vi "USB2XXXSPISlaveContinueReadTest.vi"() -> ()   [LabVIEW 2010]
panel:
  in  "stop":bool
  out "Read Data(Hex)":string
  in  "pConfig":T1
  in  "Channel Index":i32(ring) items=["SPI1_CS0", "SPI2_CS0"]
  in  "Device Index":i32(ring) items=["0", "1", "2", "3", "4", "5"]
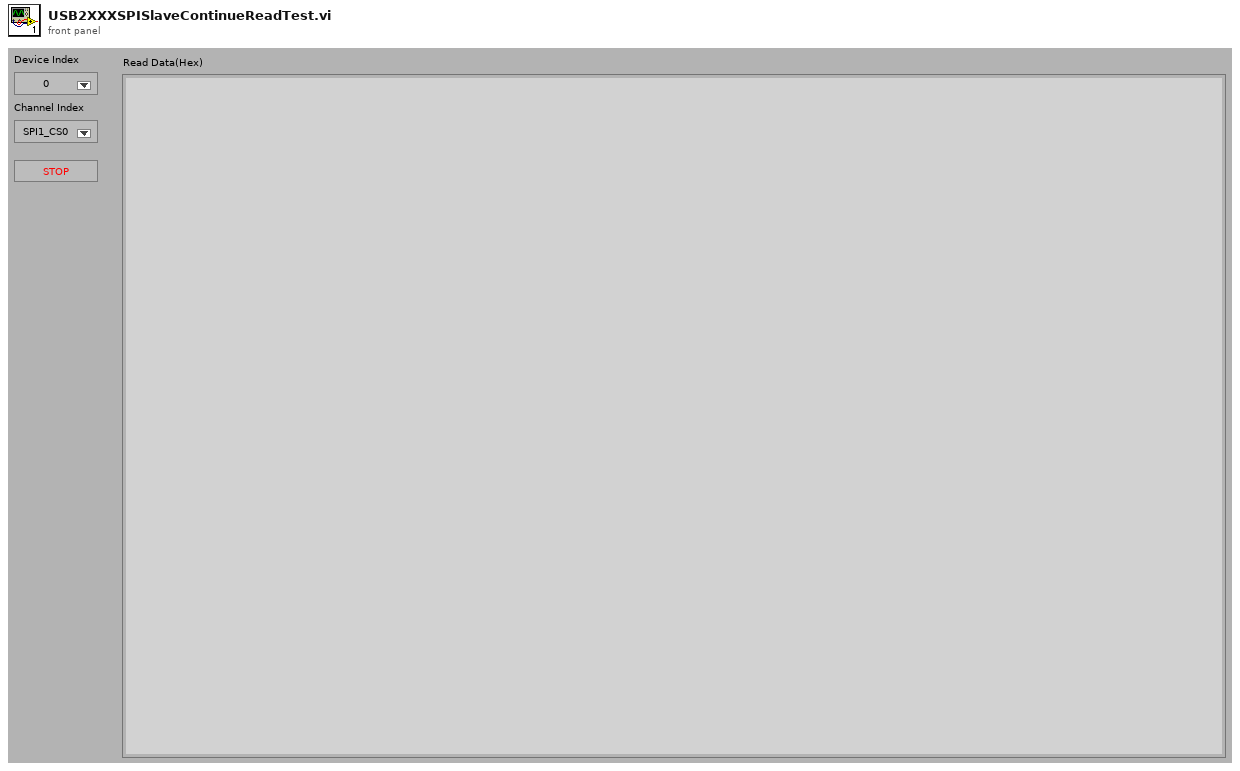
[diagram p1: front panel]
types:
  T1 = cluster{"Mode":i8, "Master":i8, "CPOL":i8, "CPHA":i8, "LSBFirst":i8, "SelPolarity":i8, "@dummy control@":i8, "@dummy control@":i8, "ClockSpeedHz":u32}
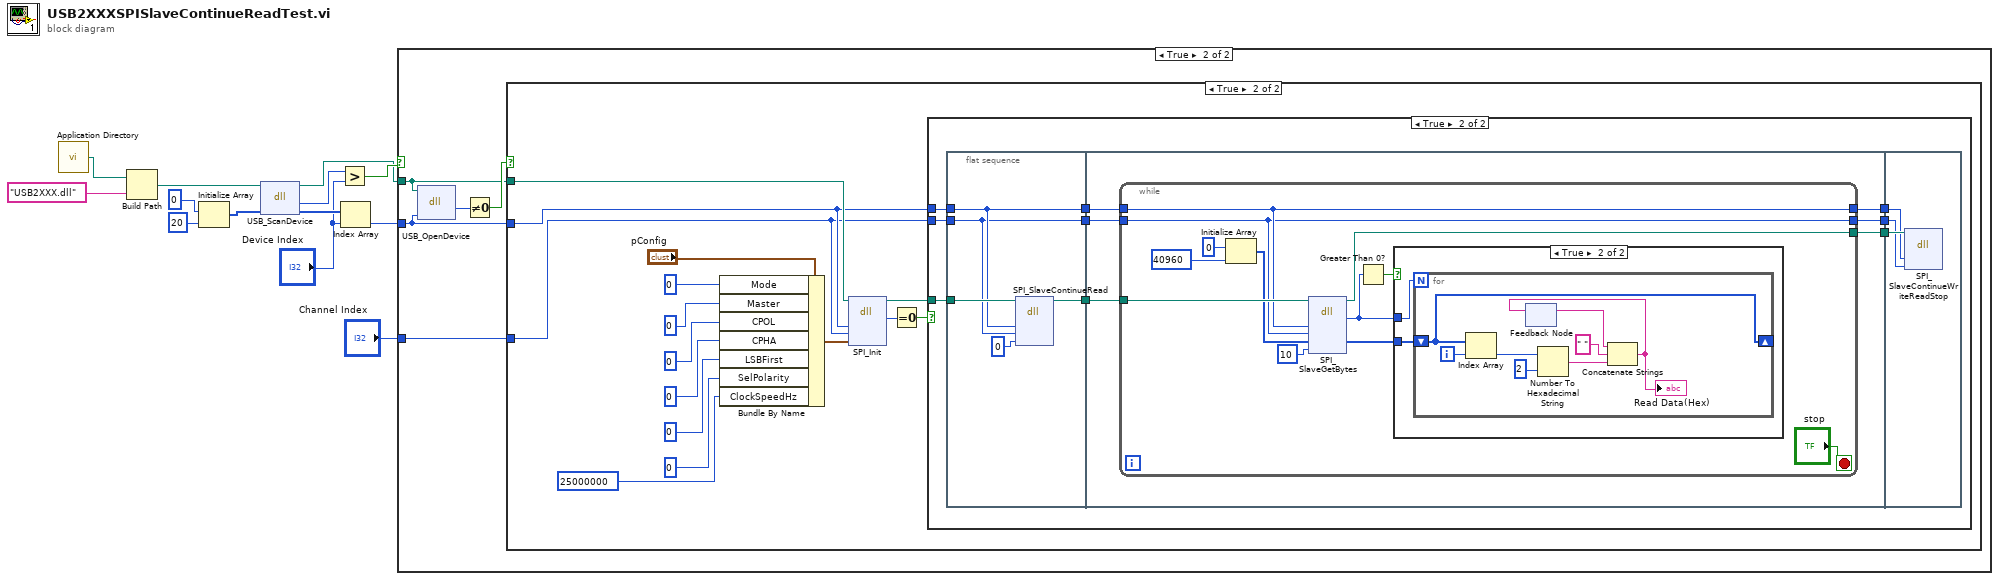
[diagram p0: block diagram]
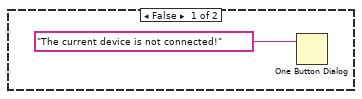
[diagram p2: hidden frame]
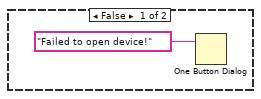
[diagram p3: hidden frame]
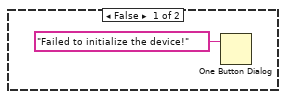
[diagram p4: hidden frame]
diagram:
  n1 = call <vilib>:"Application Directory.vi"() -> ("Application Directory"=w1:path)
  n2 = Build Path(base path=w1, name or relative path="USB2XXX.dll") -> (appended path=w2:path)
  n3 = Initialize Array(0, 20 ("dimension size")) -> (w10:i32[])
  n4 = dll-call lib="E:/OtherWork/STM32/USB2XXX_Example/trunk/Labview/PublicFiles/USB2XXX.*" fn="USB_ScanDevice"(path in=w2, "pDevNum"=w10) -> (path out=w7:path, "return type"=w9:i32, "pDevNum"=w12:i32[])  [unwired: 2 in, 1 out]
  n5 = Greater?(x=w9, y="Device Index") -> (0:w8:bool)
  n6 = Index Array(array=w12, index="Device Index") -> (element=w6:i32)
  n7 = case shown="True" w8 {
    tunnel: w7 -> [_ w17]
    tunnel: w6 -> [_ w15]
    tunnel: "Channel Index" -> [_ w16]
    frame False {
      n8 = One Button Dialog(message="The current device is not connected!") -> ()  [unwired: 1 in, 1 out]
    }
    frame True {
      n9 = dll-call lib="E:/Projects/USB2XXX_Example/sdk/api/Labview/USB2XXX.*" fn="USB_OpenDevice"(path in=w17, "DevHandle"=w15) -> ("return type"=w19:u8)  [unwired: 3 in, 2 out]
      n10 = Not Equal To 0?(x=w19) -> (x != 0?=w18:bool)
      n11 = case shown="True" w18 {
        tunnel: w17 -> [_ w26]
        tunnel: w16 -> [_ w21]
        tunnel: w15 -> [_ w22]
        frame False {
          n12 = One Button Dialog(message="Failed to open device!") -> ()  [unwired: 1 in, 1 out]
        }
        frame True {
          n13 = Bundle By Name(cluster="pConfig", "Mode"=i8 0, "Master"=i8 0, "CPOL"=i8 0, "CPHA"=i8 0, "LSBFirst"=i8 0, "SelPolarity"=i8 0, "ClockSpeedHz"=u32 25000000) -> (w27:T1)
          n14 = dll-call lib="E:/OtherWork/STM32/USB2XXX_Example/trunk/Labview/PublicFiles/USB2XXX.*" fn="SPI_Init"(path in=w26, "DevIndex"=w22, "SPIIndex"=w21, "pConfig"=w27) -> (path out=w23:path, "return type"=w25:i32)  [unwired: 5 in, 1 out]
          n15 = Equal To 0?(x=w25) -> (x = 0?=w24:bool)
          n16 = case shown="True" w24 {
            tunnel: w23 -> [_ w45]
            tunnel: w22 -> [_ w44]
            tunnel: w21 -> [_ w43]
            frame False {
              n17 = One Button Dialog(message="Failed to initialize the device!") -> ()  [unwired: 1 in, 1 out]
            }
            frame True {
              n18 = flat-sequence {
                tunnel: w45 -> [w50]
                tunnel: w44 -> [w47]
                tunnel: w43 -> [w46]
                tunnel: [w48] -> w42
                tunnel: [w47] -> w41
                tunnel: [w46] -> w40
                tunnel: w42 -> [w56]
                tunnel: w41 -> [w55]
                tunnel: w40 -> [w54]
                tunnel: [w53] -> w39
                tunnel: [w52] -> w38
                tunnel: [w51] -> w37
                tunnel: w39 -> [w81]
                tunnel: w38 -> [w80]
                tunnel: w37 -> [w79]
                frame #0 {
                  n19 = dll-call lib="E:/OtherWork/STM32/USB2XXX/trunk/USB2XXX/USB2XXX/vs2010/Release/USB2XXX.*" fn="SPI_SlaveContinueRead"(path in=w50, "DevHandle"=w47, "SPIIndex"=w46, "pSlaveReadDataHandle"=0) -> (path out=w48:path)  [unwired: 6 in, 1 out]
                }
                frame #1 {
                  n20 = while {
                    tunnel: w56 -> [w67]
                    tunnel: w55 -> [w58]
                    tunnel: w54 -> [w57]
                    tunnel: [w59] -> w53
                    tunnel: [w58] -> w52
                    tunnel: [w57] -> w51
                    stop <- "stop" stop-if-true
                    n21 = Initialize Array(u8 0 ("element"), 40960 ("element")) -> (w63:u8[])
                    n22 = dll-call lib="E:/OtherWork/STM32/USB2XXX/trunk/USB2XXX/USB2XXX/vs2010/Release/USB2XXX.*" fn="SPI_SlaveGetBytes"(path in=w67, "DevHandle"=w58, "SPIIndex"=w57, "pReadData"=w63, "TimeOutOfMs"=10) -> (path out=w59:path, "return type"=w60:i32, "pReadData"=w61:u8[])  [unwired: 5 in, 1 out]
                    n23 = Greater Than 0?(x=w60) -> (x > 0?=w62:bool)
                    n24 = case shown="True" w62 {
                      tunnel: w60 -> [_ w70]
                      tunnel: w61 -> [_ w69]
                      frame False {
                      }
                      frame True {
                        n25 = for {
                          N: w70 -> [_]
                          shift-right: [w71] -> _
                          shift-left: w69 -> [w71]
                          i -> [w78]
                          n26 = Index Array(array=w71, index=w78) -> (element=w77:u8)
                          n27 = feedback #1() -> (w75:string)  [unwired: 1 in]
                          n28 = Number To Hexadecimal String(1:i16 2 ("width (-)"), 2:w77) -> (0:w73:string)
                          n29 = Concatenate Strings(w75, " " ("string"), w73) -> (w72:string)
                          "Read Data(Hex)" <- w72
                          n30 = feedback-in #1(w72) -> ()
                        }
                      }
                    }
                  }
                }
                frame #2 {
                  n31 = dll-call lib="E:/OtherWork/STM32/USB2XXX/trunk/USB2XXX/USB2XXX/vs2010/Release/USB2XXX.*" fn="SPI_SlaveContinueWriteReadStop"(path in=w81, "DevHandle"=w80, "SPIIndex"=w79) -> ()  [unwired: 5 in, 2 out]
                }
              }
            }
          }
        }
      }
    }
  }
